vi "Locate Subset.vi"(7 "threshold y":dbl=139990.0, 8 "error in":errorcluster, 9 "Reference Channel to Split":string="B", 11 "File Path":path=path "\\\\myhome\\NHMFL/Projects/Pressure/Code/Alex/m006_092123.tdms") -> (0 "error out":errorcluster={"status"=TRUE, "code"=-2532, "source"="TDMS Read in loacate subset.vi"}, 1 "Length out":i32=2147483647, 2 "Start Index out":i32=2147483647, 3 "file path out":path=path "\\\\myhome\\NHMFL/Projects/Pressure/Code/Alex/m006_092123.tdms", 4 "Waveform Graph":waveform(dbl)[](graph))   [LabVIEW 2024]
panel:
  in  "X":string="Cryo-Con 54 (4) C"
  out "Waveform Graph 2":dbl[](graph)
  in  "Downsweep?":bool
  in  "Start":i64
  out "fractional index or x":dbl
  in  "group name in":string="p"
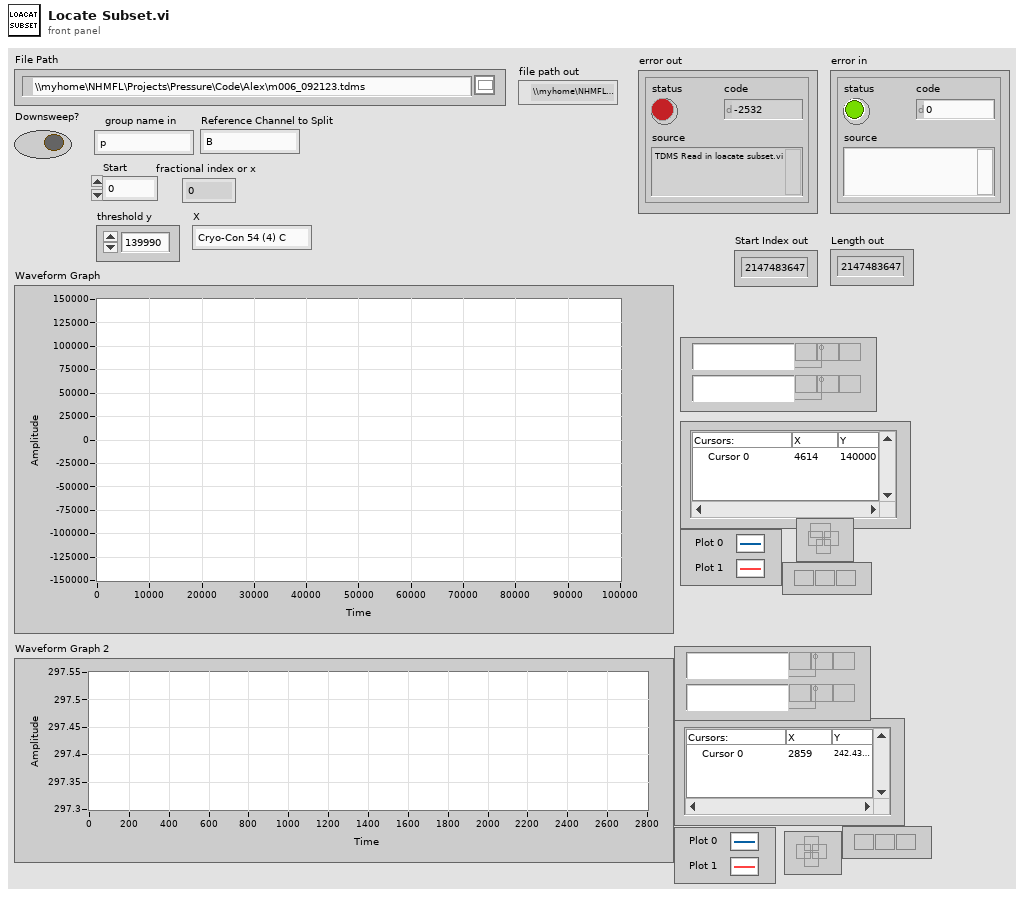
[diagram p1: front panel]
types:
  T1 = enum16{"open", "open or create", "create or replace", "create", "open (read-only)"}
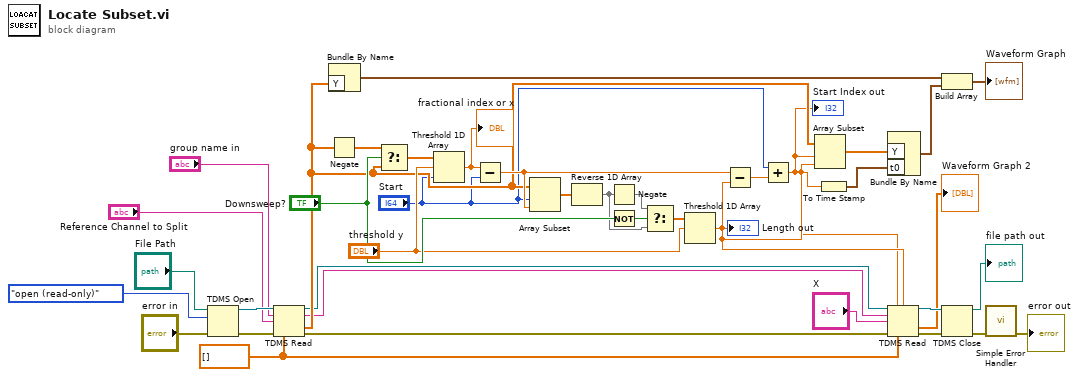
[diagram p0: block diagram]
diagram:
  w7 = dbl[] []
  n1 = TDMS Open(8:"error in", 10:T1."open (read-only)" ("operation (0:open)"), 11:"File Path") -> (0:w37:errorcluster, 3:w38:refnum<k34>)  [unwired: 4 in]
  n2 = TDMS Read(0:w38, 5:"group name in", 7:"Reference Channel to Split", 11:w37, 12:w7) -> (4:w10:refnum<k34>, 6:w8:string, 10:w14:dbl[], 15:w31:errorcluster)  [unwired: 3 in, 2 out]
  n3 = Bundle By Name("Y"=w14) -> (w34:waveform(dbl))  [unwired: 1 in]
  n4 = Negate(x=w14) -> (-x=w23:dbl[])
  n5 = Select(t=w23, s="Downsweep?", f=w14) -> (s? t:f=w24:dbl[])
  n6 = Threshold 1D Array(1:"Start", 2:"threshold y", 3:w24) -> (0:w26:dbl)
  "fractional index or x" <- w26
  n7 = Subtract(x=w26, y="Start") -> (x-y=w15:dbl)
  n8 = Array Subset(array=w14, index="Start", length=w15) -> (w22:dbl[])
  n9 = Reverse 1D Array(array=w22) -> (reversed array=w18:dbl[])
  n10 = Negate(x=w18) -> (-x=w19:dbl[])
  n11 = Not(x="Downsweep?") -> (.not. x?=w20:bool)
  n12 = Select(t=w19, s=w20, f=w18) -> (s? t:f=w17:dbl[])
  n13 = Threshold 1D Array(2:"threshold y", 3:w17) -> (0:w3:dbl)  [unwired: 1 in]
  "Length out" <- w3
  n14 = Subtract(x=w15, y=w3) -> (x-y=w13:dbl)
  n15 = Add(x="Start", y=w13) -> (x+y=w1:dbl)
  "Start Index out" <- w1
  n16 = Array Subset(array=w14, index=w1, length=w3) -> (w12:dbl[])
  n17 = To Time Stamp(1:w1) -> (0:w2:timestamp)
  n18 = Bundle By Name("Y"=w12, "t0"=w2) -> (w33:waveform(dbl))  [unwired: 1 in]
  n19 = TDMS Read(0:w10, 1:w1, 2:w3, 5:w8, 7:"X", 11:w31, 12:w7) -> (4:w9:refnum<k34>, 10:→"Waveform Graph 2":dbl[], 15:w11:errorcluster)  [unwired: 1 in, 3 out]
  n20 = Build Array(w34, w33) -> (→"Waveform Graph":waveform(dbl)[])
  n21 = TDMS Close(8:w11, 11:w9) -> (0:w29:errorcluster, 3:→"file path out":path)
  n22 = call <vilib>:"Simple Error Handler.vi"("error in (no error)"=w29) -> ("error out"=→"error out":errorcluster)  [unwired: 4 in, 4 out]
